vi "Global 3.vi"() -> ()   [LabVIEW 2020]
panel:
  in  "Byte Stream File Refnum":refnum<file>
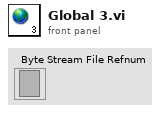
[diagram p1: front panel]
diagram:
